vi "压装试验判定.vi"(7 "Result":refnum<vi>, 10 "判定参数":T1, 11 "XY曲线":cluster{"X":dbl[], "Y":dbl[]}[](array[cluster])) -> (2 "判定项长度":i32, 3 "OK？":bool)   [LabVIEW 2020]
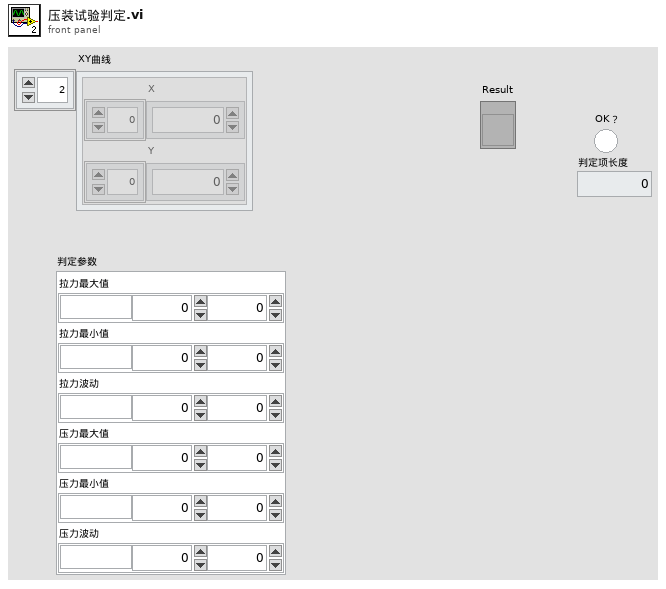
[diagram p1: front panel]
types:
  T1 = cluster{"拉力最大值":cluster{"单位":string, "下限":dbl, "上限":dbl}, "拉力最小值":cluster{"单位":string, "下限":dbl, "上限":dbl}, "拉力波动":cluster{"单位":string, "下限":dbl, "上限":dbl}, "压力最大值":cluster{"单位":string, "下限":dbl, "上限":dbl}, "压力最小值":cluster{"单位":string, "下限":dbl, "上限":dbl}, "压力波动":cluster{"单位":string, "下限":dbl, "上限":dbl}}
  T2 = cluster{"位移":cluster{"单位":string, "下限":dbl, "上限":dbl}, "拉力":cluster{"单位":string, "下限":dbl, "上限":dbl}, "位移1":cluster{"单位":string, "下限":dbl, "上限":dbl}, "压力":cluster{"单位":string, "下限":dbl, "上限":dbl}}
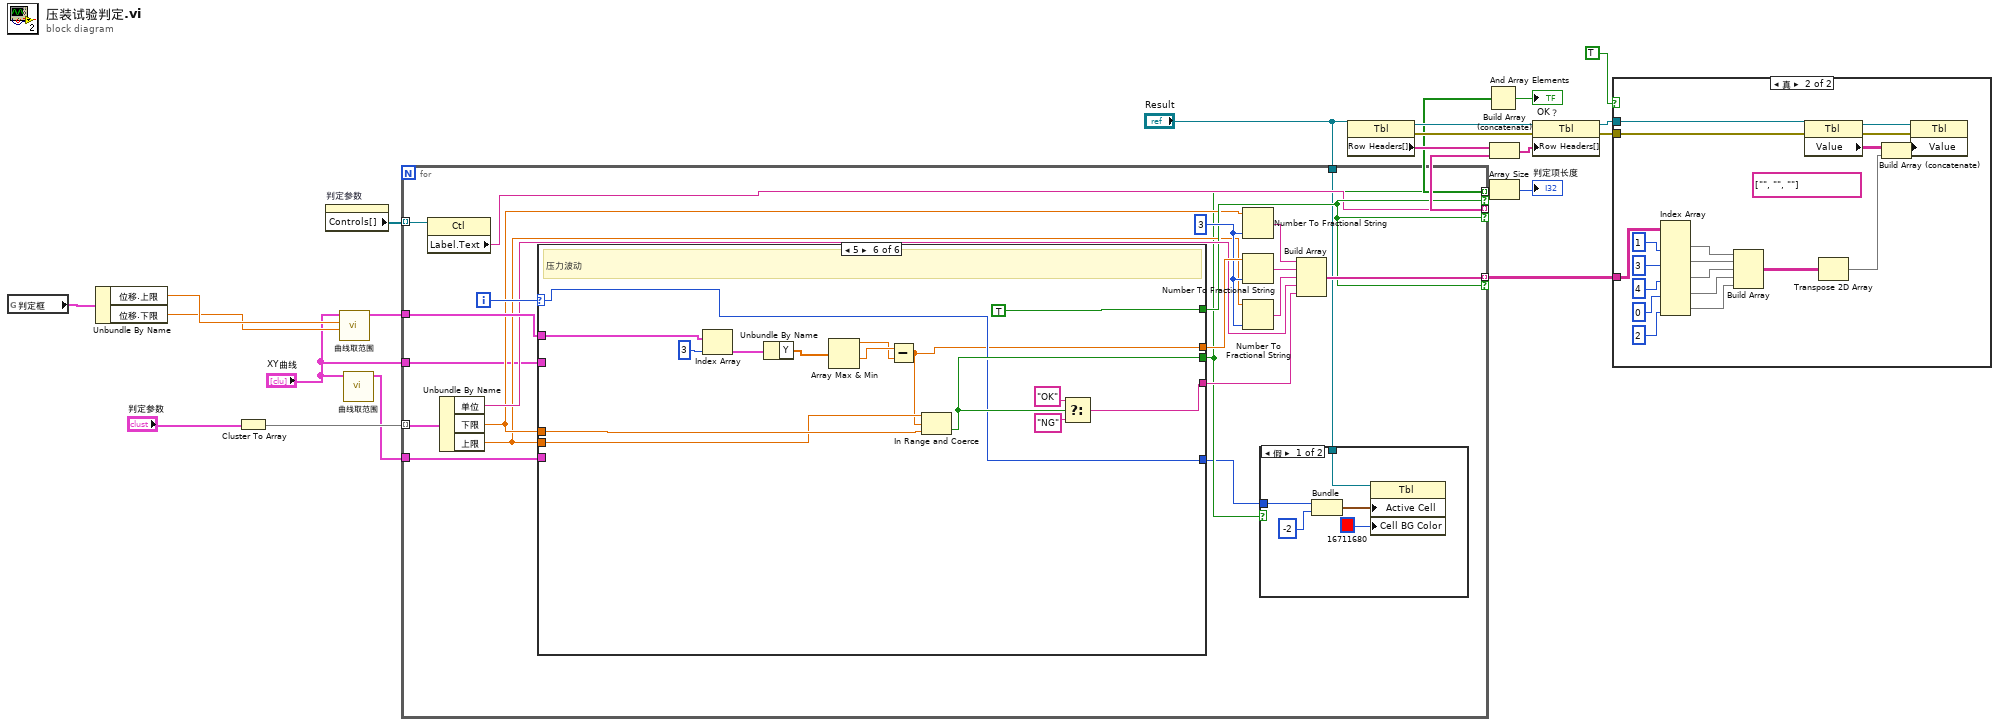
[diagram p0: block diagram]
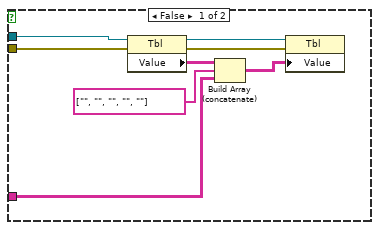
[diagram p2: hidden frame]
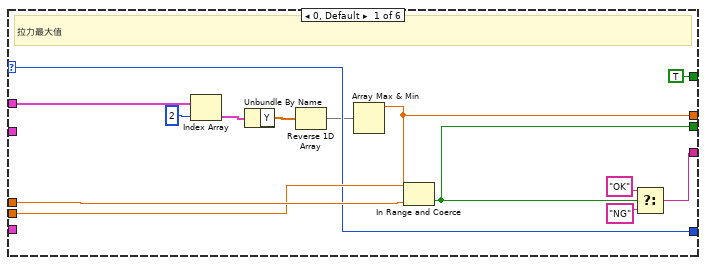
[diagram p4: hidden frame]
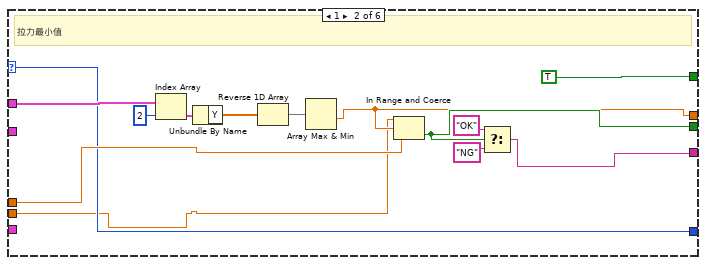
[diagram p5: hidden frame]
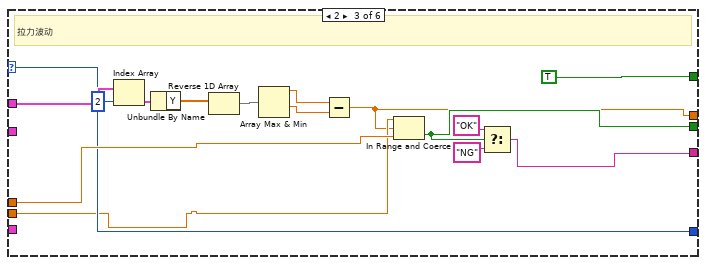
[diagram p6: hidden frame]
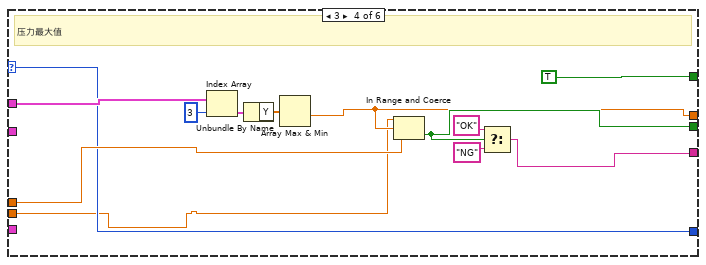
[diagram p7: hidden frame]
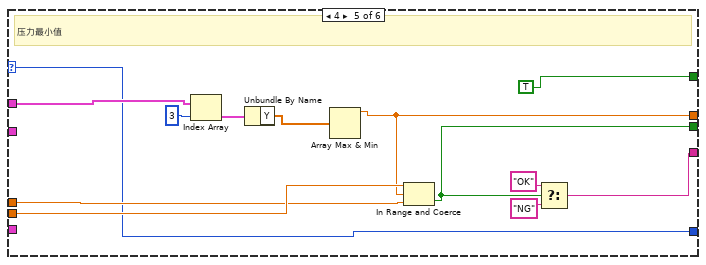
[diagram p8: hidden frame]
diagram:
  n1 = global read "判定参数.vi" "判定框"() -> (w4:T2)
  n2 = Unbundle By Name(w4) -> ("位移.上限"=w6:dbl, "位移.下限"=w5:dbl)
  n3 = Cluster To Array(cluster="判定参数") -> (array=w22:cluster{"单位":string, "下限":dbl, "上限":dbl}[])
  n4 = property on="判定参数" class="Clust (严格)"() -> ("Controls[]"=w12:refnum<vi>[])  [unwired: 2 in, 2 out]
  n5 = call "曲线取范围.vi"("下限"=w5, "上限"=w6, "曲线In"="XY曲线") -> ("曲线Out"=w8:cluster{"X":dbl[], "Y":dbl[]}[])  [unwired: 8 in]
  n6 = call "曲线取范围.vi"("曲线In"="XY曲线") -> ("曲线Out"=w2:cluster{"X":dbl[], "Y":dbl[]}[])  [unwired: 10 in]
  n7 = for {
    tunnel: w22 -> [w43] mode=indexing
    tunnel: w12 -> [w41] mode=indexing
    tunnel: w8 -> [w39]
    tunnel: [w24] -> w10 mode=indexing if=w31
    tunnel: [w32] -> w13 mode=indexing if=w31
    tunnel: [w28] -> w15 mode=indexing if=w31
    tunnel: "XY曲线" -> [w27]
    tunnel: w2 -> [w26]
    tunnel: "Result" -> [w25]
    i -> [w42]
    w38 = i16 3 ("精度(6)")
    n8 = property class="Ctl"(reference=w41) -> ("Label.Text"=w28:string)  [unwired: 1 in, 2 out]
    n9 = Unbundle By Name(w43) -> ("单位"=w33:string, "下限"=w30:dbl, "上限"=w29:dbl)
    n10 = case shown="5" w42 {
      selector: w42 -> [w52 w71 w87 w100 w107 w127]
      tunnel: [w50 w70 w77 w99 w106 w121] -> w40
      tunnel: w39 -> [w62 w76 w92 w105 w115 w130]
      tunnel: [w57 w75 w91 w104 w118 w133] -> w34
      tunnel: [w56 w74 w90 w103 w117 w132] -> w24
      tunnel: w30 -> [w55 w73 w89 w102 w114 w129]
      tunnel: w29 -> [w54 w69 w86 w98 w116 w128]
      tunnel: [TRUE TRUE TRUE TRUE TRUE TRUE] -> w31
      tunnel: w27 -> [_ _ _ _ _ _]
      tunnel: w26 -> [_ _ _ _ _ _]
      tunnel: [w52 w71 w87 w100 w107 w127] -> w23
      frame 0, Default {
        # "拉力最大值"
        n11 = Index Array(array=w62, index=2 ("索引")) -> (element=w60:cluster{"X":dbl[], "Y":dbl[]})
        n12 = Unbundle By Name(w60) -> ("Y"=w51:dbl[])
        n13 = Reverse 1D Array(array=w51) -> (reversed array=w49:dbl[])
        n14 = Array Max & Min(array=w49) -> (max value=w50:dbl)  [unwired: 3 out]
        n15 = In Range and Coerce(upper limit=w54, x=w50, lower limit=w55) -> (In Range?=w56:bool)  [unwired: 1 out]
        n16 = Select(t="OK", s=w56, f="NG") -> (s? t:f=w57:string)
      }
      frame 1 {
        # "拉力最小值"
        n17 = Index Array(array=w76, index=2 ("索引")) -> (element=w68:cluster{"X":dbl[], "Y":dbl[]})
        n18 = Unbundle By Name(w68) -> ("Y"=w65:dbl[])
        n19 = Reverse 1D Array(array=w65) -> (reversed array=w63:dbl[])
        n20 = Array Max & Min(array=w63) -> (min value=w70:dbl)  [unwired: 3 out]
        n21 = In Range and Coerce(upper limit=w69, x=w70, lower limit=w73) -> (In Range?=w74:bool)  [unwired: 1 out]
        n22 = Select(t="OK", s=w74, f="NG") -> (s? t:f=w75:string)
      }
      frame 2 {
        # "拉力波动"
        n23 = Index Array(array=w92, index=2 ("索引")) -> (element=w85:cluster{"X":dbl[], "Y":dbl[]})
        n24 = Unbundle By Name(w85) -> ("Y"=w82:dbl[])
        n25 = Reverse 1D Array(array=w82) -> (reversed array=w80:dbl[])
        n26 = Array Max & Min(array=w80) -> (max value=w79:dbl, min value=w78:dbl)  [unwired: 2 out]
        n27 = Subtract(x=w79, y=w78) -> (x-y=w77:dbl)
        n28 = In Range and Coerce(upper limit=w86, x=w77, lower limit=w89) -> (In Range?=w90:bool)  [unwired: 1 out]
        n29 = Select(t="OK", s=w90, f="NG") -> (s? t:f=w91:string)
      }
      frame 3 {
        # "压力最大值"
        n30 = Index Array(array=w105, index=3 ("索引")) -> (element=w97:cluster{"X":dbl[], "Y":dbl[]})
        n31 = Unbundle By Name(w97) -> ("Y"=w94:dbl[])
        n32 = Array Max & Min(array=w94) -> (min value=w99:dbl)  [unwired: 3 out]
        n33 = In Range and Coerce(upper limit=w98, x=w99, lower limit=w102) -> (In Range?=w103:bool)  [unwired: 1 out]
        n34 = Select(t="OK", s=w103, f="NG") -> (s? t:f=w104:string)
      }
      frame 4 {
        # "压力最小值"
        n35 = Index Array(array=w115, index=3 ("索引")) -> (element=w109:cluster{"X":dbl[], "Y":dbl[]})
        n36 = Unbundle By Name(w109) -> ("Y"=w108:dbl[])
        n37 = Array Max & Min(array=w108) -> (max value=w106:dbl)  [unwired: 3 out]
        n38 = In Range and Coerce(upper limit=w116, x=w106, lower limit=w114) -> (In Range?=w117:bool)  [unwired: 1 out]
        n39 = Select(t="OK", s=w117, f="NG") -> (s? t:f=w118:string)
      }
      frame 5 {
        # "压力波动"
        n40 = Index Array(array=w130, index=3 ("索引")) -> (element=w123:cluster{"X":dbl[], "Y":dbl[]})
        n41 = Unbundle By Name(w123) -> ("Y"=w122:dbl[])
        n42 = Array Max & Min(array=w122) -> (max value=w119:dbl, min value=w120:dbl)  [unwired: 2 out]
        n43 = Subtract(x=w120, y=w119) -> (x-y=w121:dbl)
        n44 = In Range and Coerce(upper limit=w128, x=w121, lower limit=w129) -> (In Range?=w132:bool)  [unwired: 1 out]
        n45 = Select(t="OK", s=w132, f="NG") -> (s? t:f=w133:string)
      }
    }
    n46 = Number To Fractional String(number=w30, precision (6)=w38) -> (F-format string=w37:string)  [unwired: 2 in]
    n47 = Number To Fractional String(number=w40, precision (6)=w38) -> (F-format string=w36:string)  [unwired: 2 in]
    n48 = Number To Fractional String(number=w29, precision (6)=w38) -> (F-format string=w35:string)  [unwired: 2 in]
    n49 = case shown="假" w24 {
      tunnel: w25 -> [w48 _]
      tunnel: w23 -> [w44 _]
      frame False {
        n50 = Bundle(w44, "索引"=-2) -> (w45:cluster{i32, "索引":i32})  [unwired: 1 in]
        n51 = property class="Tbl"(reference=w48, "Active Cell"=w45, "Cell BG Color"=u32 16711680 ("活动单元格:单元格背景色")) -> ()  [unwired: 1 in, 2 out]
      }
      frame True {
      }
    }
    n52 = Build Array(w37, w36, w35, w33, w34) -> (w32:string[])
  }
  n53 = property class="Tbl"(reference="Result") -> (reference out=w17:refnum<vi>, error out=w20:errorcluster, "Row Headers[]"=w14:string[])  [unwired: 1 in]
  n54 = And Array Elements(Boolean array=w10) -> (logical AND=→"OK？":bool)
  n55 = Build Array (concatenate)(w14, w15) -> (w16:string[])
  n56 = Array Size(array=w10) -> (size(s)=→"判定项长度":i32)
  n57 = property class="Tbl"(reference=w17, error in=w20, "Row Headers[]"=w16) -> (reference out=w18:refnum<vi>, error out=w19:errorcluster)
  n58 = case shown="真" TRUE {
    tunnel: w19 -> [w139 w158]
    tunnel: w18 -> [w136 w155]
    tunnel: w13 -> [w135 w154]
    frame False {
      n59 = property class="Tbl"(reference=w136, error in=w139) -> (reference out=w137:refnum<vi>, error out=w138:errorcluster, "Value"=w140:string[][])
      n60 = Build Array (concatenate)(w140, string[] ["", "", "", "", ""], w135) -> (w141:string[][])
      n61 = property class="Tbl"(reference=w137, error in=w138, "Value"=w141) -> ()  [unwired: 2 out]
    }
    frame True {
      (unwired) string[] ["", "", ""]
      n62 = Index Array(array=w154, index (col) #1=1 ("禁用的索引 (列)"), index (col) #2=3 ("索引 (列)"), index (col) #3=4 ("索引 (列)"), index (col) #4=0 ("索引 (列)"), index (col) #5=2 ("索引 (列)")) -> (element #1=w150:string[], element #2=w149:string[], element #3=w148:string[], element #4=w143:string[], element #5=w142:string[])  [unwired: 5 in]
      n63 = Build Array(w150, w149, w148, w143, w142) -> (w147:string[][])
      n64 = property class="Tbl"(reference=w155, error in=w158) -> (reference out=w156:refnum<vi>, error out=w157:errorcluster, "Value"=w159:string[][])
      n65 = Transpose 2D Array(2D array=w147) -> (transposed array=w146:string[][])
      n66 = Build Array (concatenate)(w159, w146) -> (w160:string[][])
      n67 = property class="Tbl"(reference=w156, error in=w157, "Value"=w160) -> ()  [unwired: 2 out]
    }
  }
